vi "Store Tree Appearance.vi"(8 "Error In":errorcluster, 11 "State In":T1) -> (0 "Error Out":errorcluster, 3 "State Out":T1)   [LabVIEW 2018, in "Bookmark Manager.lvlib"]
uses:
  Bookmark Manager.lvlib
  Controls/State.ctl
  <vilib>/addons/analyzer/_analyzerctrls.llb/VIAnCtl Analysis App Info.ctl
  Controls/Bookmark.ctl
  Controls/VI Identifier.ctl
  Controls/Bookmarks Groups.ctl
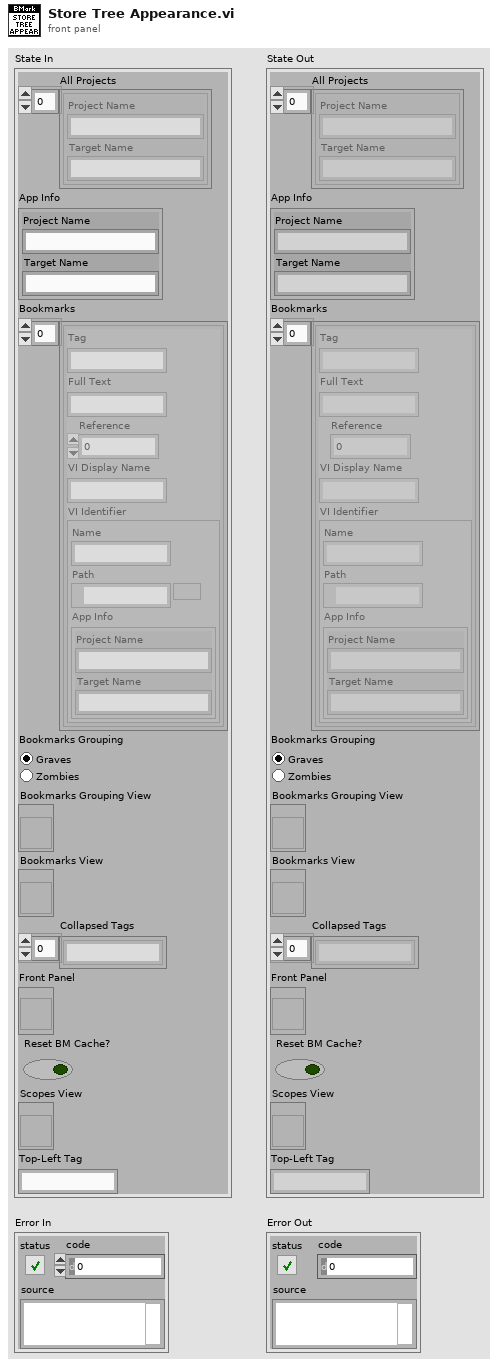
[diagram p1: front panel]
types:
  T1 = typedef "Bookmark Manager.lvlib/State.ctl" = cluster{"All Projects":T2[], "App Info":T2, "Bookmarks":T3[], "Bookmarks Grouping":T5, "Bookmarks Grouping View":refnum<vi>, "Bookmarks View":refnum<vi>, "Collapsed Tags":string[], "Front Panel":refnum<vi>, "Reset BM Cache?":bool, "Scopes View":refnum<vi>, "Top-Left Tag":string}
  T2 = typedef "VIAnCtl Analysis App Info.ctl" = cluster{"Project Name":string, "Target Name":string}
  T3 = typedef "Bookmark Manager.lvlib/Bookmark.ctl" = cluster{"Tag":string, "Full Text":string, "Reference":i32, "VI Display Name":string, "VI Identifier":T4}
  T4 = typedef "Bookmark Manager.lvlib/VI Identifier.ctl" = cluster{"Name":string, "Path":path, "App Info":T2}
  T5 = typedef "Bookmark Manager.lvlib/Bookmarks Groups.ctl" = enum32{"Graves", "Zombies"}
  T6 = typedef "LVNodeAndColumnTypeDef.ctl" = cluster{"Node":string, "Column":i32}
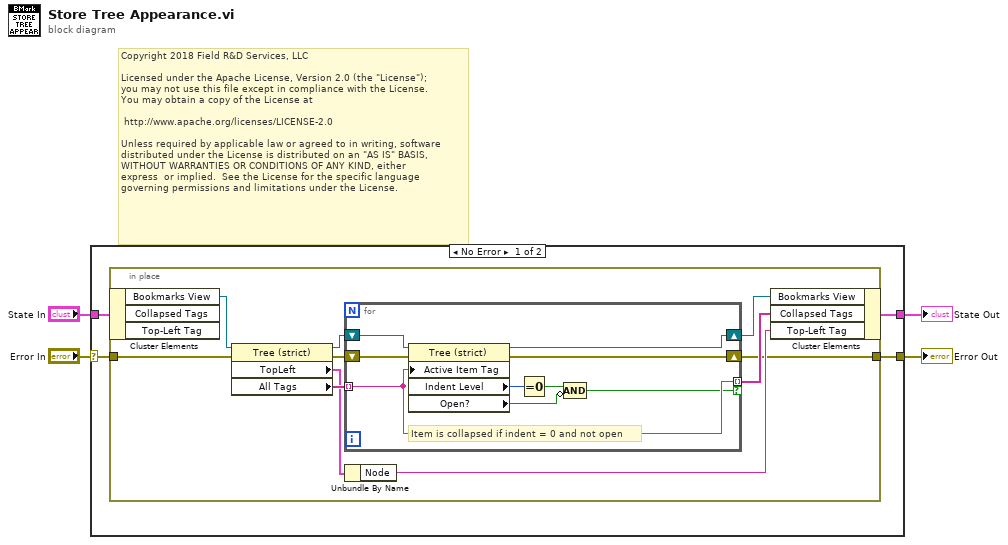
[diagram p0: block diagram]
diagram:
  # "Copyright 2018 Field R&D Services, LLC\n\nLicensed under the Apache License, Version 2.0 (the \"License\");\nyou may not use this file except in compliance with the License.\nYou may obtain a copy of the License at\n\n\thttp://www.apache.org/licenses/LICENSE-2.0\n\nUnless required by applicable law or agreed to in writing, software\ndistributed under the License is distributed on an \"AS IS\" BASIS,\nWITHOUT WARRANTIES OR CONDITIONS OF ANY KIND, either \nexpress  or implied.  See the License for the specific language \ngoverning permissions and limitations under the License."
  n1 = case shown="No Error" "Error In" {
    selector: "Error In" -> [w5 w28]
    tunnel: [w8 w28] -> w4
    tunnel: [w7 w29] -> w3
    tunnel: "State In" -> [w6 w29]
    frame No Error {
      n2 = in-place {
        in-place-border: w5 -> [w17]
        in-place-border: [w9] -> w8
        n3 = in-place-cluster #1(w6) -> ("Bookmarks View"=w18:refnum<vi>)  [unwired: 2 out]
        n4 = property class="Tree (strict)"(reference=w18, error in=w17) -> (reference out=w16:refnum<vi>, error out=w14:errorcluster, "TopLeft"=w11:T6, "All Tags"=w15:string[])
        n5 = for {
          tunnel: w15 -> [w26] mode=indexing
          tunnel: [w26] -> w13 mode=indexing if=w22
          shift-right: [w21] -> w12
          shift-left: w16 -> [w27]
          shift-right: [w19] -> w9
          shift-left: w14 -> [w20]
          # "Item is collapsed if indent = 0 and not open"
          n6 = property class="Tree (strict)"(reference=w27, error in=w20, "Active Item Tag"=w26) -> (reference out=w21:refnum<vi>, error out=w19:errorcluster, "Indent Level"=w24:i32, "Open?"=w23:bool)
          n7 = Equal To 0?(x=w24) -> (x = 0?=w25:bool)
          n8 = Compound Arithmetic op=AND(w25, invert w23) -> (w22:bool)
        }
        n9 = Unbundle By Name(w11) -> ("Node"=w10:string)
        n10 = in-place-cluster #1("Bookmarks View"=w12, "Collapsed Tags"=w13, "Top-Left Tag"=w10) -> (w7:T1)
      }
    }
    frame Error {
    }
  }
  "Error Out" <- w4
  "State Out" <- w3
